vi "Multiple Analog Waveforms Output Generator LV2012.vi"() -> ()   [LabVIEW 2020]
uses:
  <vilib>/Utility/error.llb/DialogType.ctl
  <vilib>/DAQmx/write.llb/DAQmx Write (Analog 1D Wfm NChan NSamp).vi
  <vilib>/DAQmx/create/channels.llb/DAQmx Create Channel (AO-Voltage-Basic).vi
  <vilib>/DAQmx/configure/timing.llb/DAQmx Timing (Sample Clock).vi
  <vilib>/DAQmx/miscellaneous.llb/DAQmx Fill In Error Info.vi
  <resource>/objmgr/daqmx.rc
  <vilib>/measure/NI_MABase.lvlib
panel:
  in  "Phase (Deg)":dbl[](array[numeric])
  in  "Waveform Type":T1(array[ring])
  in  "Desired Frequency":dbl[](array[numeric]) caption="Desired Frequency (Hz)"
  in  "Amplitude":dbl[](array[numeric]) caption="Amplitude (V)"
  in  "Sample Clock Rate":dbl=10000.0 format="%.2f"
  in  "Samples per Buffer":dbl=1000.0
  in  "Physical Channels":tag="NI-USB6343/ao0:3"
  in  "Minimum Value":dbl=-10.0 format="%0.2f"
  in  "Maximum Value":dbl=10.0 format="%0.2f"
  out "Output Data":waveform(dbl)[](graph)
  in  "stop":bool
  # "Overview: This application demonstrates a method for generating multiple analog waveforms output on multiple channels. It also integrates a method for dynamically varying the output waveform attributes. All parameters including the waveform type, may be updated at run-time. This example is scalable to any number of available channels available on the system.\nRequirements: LabVIEW Full Developement System\nInstruction:\n1. Configure the physical channel.\n2. Configure the waveform attributes.\n3. Run the VI."
  # "DAQmx Task Configuration"
  # "Waveform Attributes"
  # "Introduction: \nThis application demonstrates a method\nfor generating multiple analog waveforms\noutput on multiple channels. It also integrates \na method for dynamically varying the output \nwaveform attributes. All parameters including \nthe waveform type, may be updated at run-\ntime. This example is scalable to any number \nof available channels."
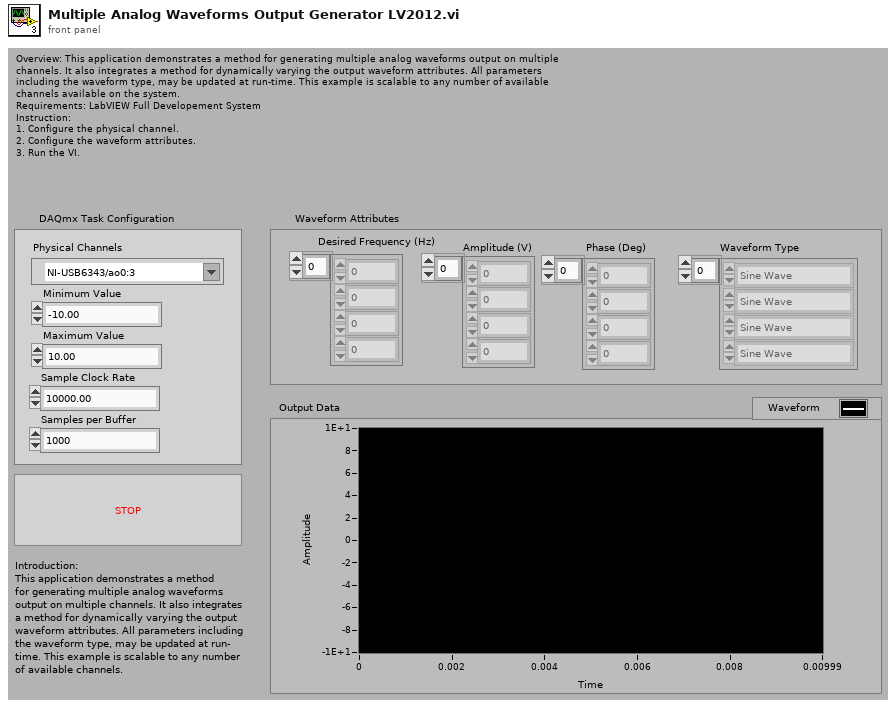
[diagram p1: front panel]
types:
  T1 = enum16{"Sine Wave", "Triangle Wave", "Square Wave", "Sawtooth Wave"}[]
  T2 = typedef "DialogType.ctl" = u16
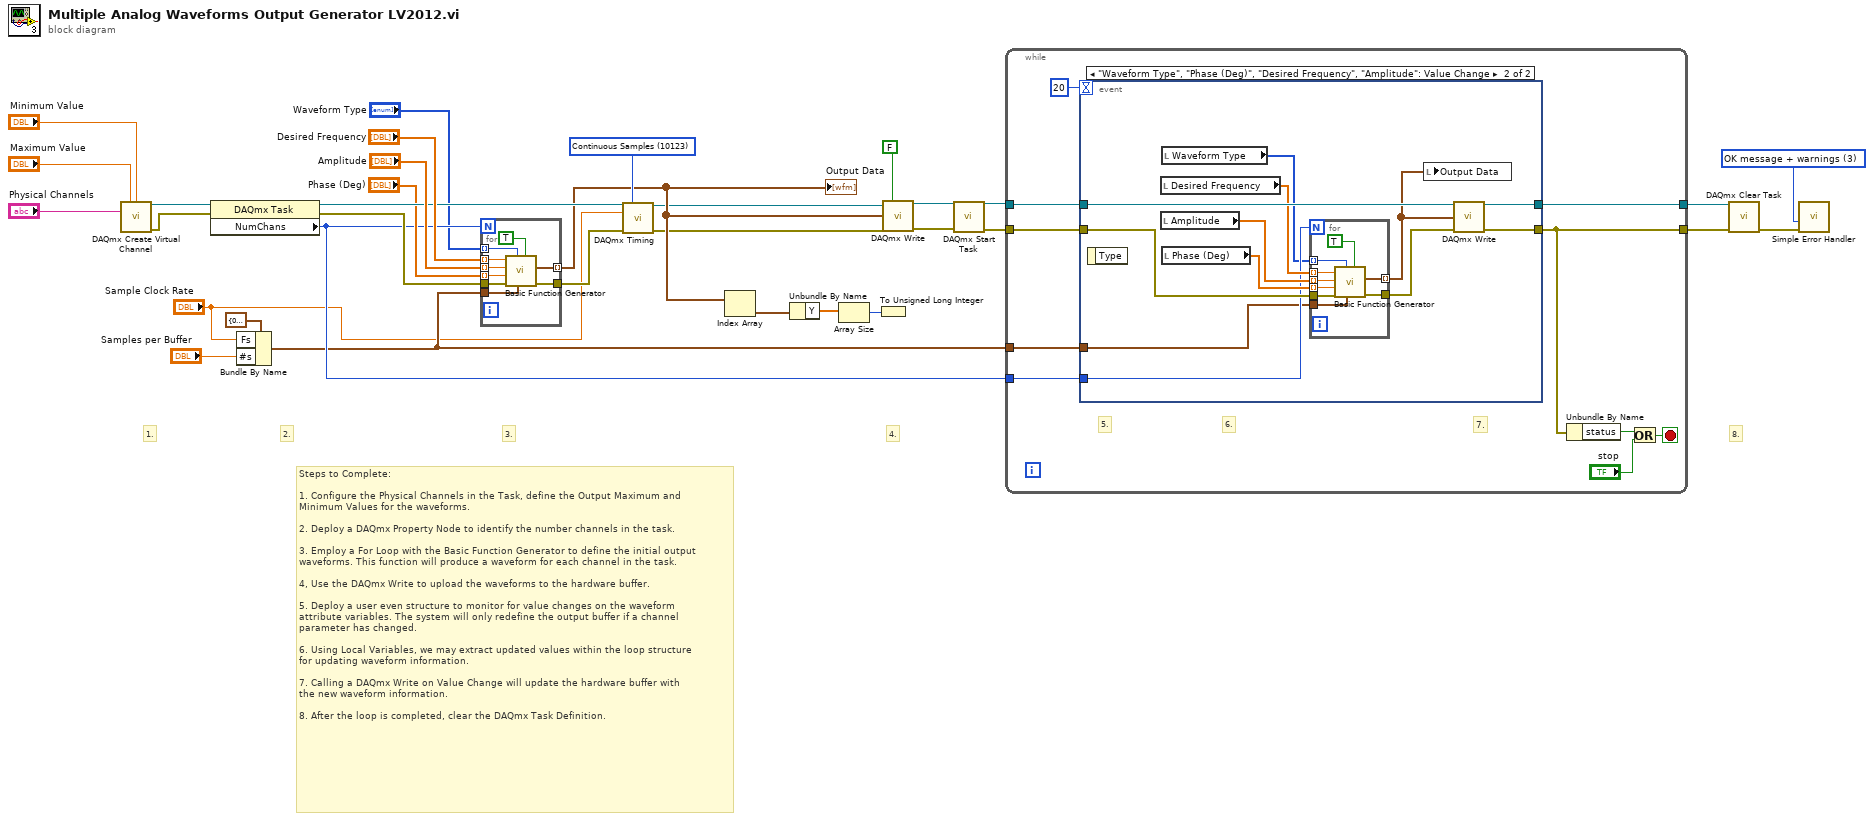
[diagram p0: block diagram]
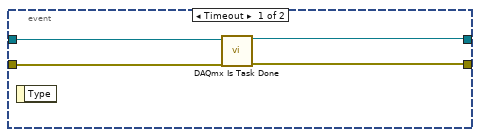
[diagram p2: hidden frame]
diagram:
  w24 = T2 3 items=["no dialog", "OK message", "continue or stop message", "OK message + warnings", "continue/stop + warnings"] ("type of dialog (OK msg:1)")
  w31 = 10123 items=["Finite Samples"=10178, "Continuous Samples"=10123] ("sample mode")
  # "Steps to Complete:\n\n1. Configure the Physical Channels in the Task, define the Output Maximum and \nMinimum Values for the waveforms. \n\n2. Deploy a DAQmx Property Node to identify the number channels in the task. \n\n3. Employ a For Loop with the Basic Function Generator to define the initial output\nwaveforms. This function will produce a waveform for each channel in the task. \n\n4, Use the DAQmx Write to upload the waveforms to the hardware buffer. \n\n5. Deploy a user even structure to monitor for value changes on the waveform \nattribute variables. The system will only redefine the output buffer if a channel \nparameter has changed. \n\n6. Using Local Variables, we may extract updated values within the loop structure\nfor updating waveform information. \n\n7. Calling a DAQmx Write on Value Change will update the hardware buffer with\nthe new waveform information. \n\n8. After the loop is completed, clear the DAQmx Task Definition."
  # "8."
  # "4."
  # "3."
  # "2."
  # "1."
  n1 = call-poly <vilib>:"DAQmx Create Virtual Channel.vi"("maximum value"="Maximum Value", "minimum value"="Minimum Value", "physical channels"="Physical Channels") -> ("task out"=w18:refnum<k21>, "error out"=w15:errorcluster)  [unwired: 11 in]
  n2 = property class="DAQmx Task"(reference=w18, error in=w15) -> (reference out=w17:refnum<k21>, error out=w16:errorcluster, "NumChans"=w13:u32)
  n3 = Bundle By Name(cluster=cluster{"Fs":dbl, "#s":dbl} {"Fs"=0.0, "#s"=0.0} ("sampling info"), "Fs"="Sample Clock Rate", "#s"="Samples per Buffer") -> (w9:cluster{"Fs":dbl, "#s":dbl})
  n4 = for {
    N: w13 -> [_]
    tunnel: "Amplitude" -> [w42] mode=indexing
    tunnel: "Desired Frequency" -> [w41] mode=indexing
    tunnel: [w40] -> w19
    tunnel: w16 -> [w39]
    tunnel: [w38] -> w6 mode=indexing
    tunnel: "Phase (Deg)" -> [w37] mode=indexing
    tunnel: w9 -> [w35]
    tunnel: "Waveform Type" -> [w34] mode=indexing
    n5 = call <vilib>:"Basic Function Generator.vi"("reset signal"=TRUE, "sampling info"=w35, "signal type"=w34, "error in (no error)"=w39, "phase"=w37, "amplitude"=w42, "frequency"=w41) -> ("error out"=w40:errorcluster, "signal out"=w38:waveform(dbl))  [unwired: 2 in, 1 out]
  }
  "Output Data" <- w6
  n6 = call-poly <vilib>:"DAQmx Timing.vi"("task/channels in"=w17, "sample mode"=w31, "rate"="Sample Clock Rate", "error in"=w19) -> ("task out"=w1:refnum<k21>, "error out"=w2:errorcluster)  [unwired: 10 in]
  n7 = Index Array(array=w6) -> (element=w5:waveform(dbl))  [unwired: 1 in]
  n8 = Unbundle By Name(w5) -> ("Y"=w4:dbl[])
  n9 = Array Size(array=w4) -> (size(s)=w3:i32)
  n10 = To Unsigned Long Integer(number=w3) -> ()  [unwired: 1 out]
  n11 = call-poly <vilib>:"DAQmx Write.vi"("task/channels in"=w1, "auto start"=FALSE, "data"=w6, "error in"=w2) -> ("task out"=w28:refnum<k21>, "error out"=w27:errorcluster)  [unwired: 9 in, 1 out]
  n12 = call <vilib>:"DAQmx Start Task.vi"("task/channels in"=w28, "error in"=w27) -> ("task out"=w32:refnum<k21>, "error out"=w26:errorcluster)  [unwired: 12 in]
  n13 = while {
    tunnel: w32 -> [w49]
    tunnel: w26 -> [w48]
    tunnel: w9 -> [w47]
    tunnel: w13 -> [w46]
    tunnel: [w45] -> w12
    tunnel: [w44] -> w11
    stop <- w51 stop-if-true
    # "7."
    # "6."
    # "5."
    n14 = event shown="[1] \"Waveform Type\", \"Phase (Deg)\", \"Desired Frequency\", \"Amplitude\": Value Change" {
      selector: _ -> [_ _]
      dyn-events: _ -> [_ _]
      timeout: 20 -> [_ _]
      tunnel: w49 -> [w56 w68]
      tunnel: w48 -> [w55 w67]
      tunnel: w47 -> [_ w58]
      tunnel: [w54 w62] -> w45
      tunnel: [w53 w61] -> w44
      tunnel: w46 -> [_ w59]
      event Timeout {
        n15 = event-data() -> ()  [unwired: 1 in, 1 out]
        n16 = call <vilib>:"DAQmx Is Task Done.vi"("task/channels in"=w56, "error in"=w55) -> ("task out"=w54:refnum<k21>, "error out"=w53:errorcluster)  [unwired: 11 in, 1 out]
      }
      event "Waveform Type", "Phase (Deg)", "Desired Frequency", "Amplitude": Value Change {
        n17 = event-data() -> ()  [unwired: 1 in, 1 out]
        n18 = local read "Desired Frequency"() -> (w65:dbl[])
        n19 = local read "Amplitude"() -> (w64:dbl[])
        n20 = local read "Waveform Type"() -> (w57:T1)
        n21 = local read "Phase (Deg)"() -> (w63:dbl[])
        n22 = for {
          N: w59 -> [_]
          tunnel: [w77] -> w66
          tunnel: [w76] -> w60 mode=indexing
          tunnel: w67 -> [w75]
          tunnel: w65 -> [w74] mode=indexing
          tunnel: w64 -> [w73] mode=indexing
          tunnel: w63 -> [w72] mode=indexing
          tunnel: w58 -> [w70]
          tunnel: w57 -> [w69] mode=indexing
          n23 = call <vilib>:"Basic Function Generator.vi"("reset signal"=TRUE, "sampling info"=w70, "signal type"=w69, "error in (no error)"=w75, "phase"=w72, "amplitude"=w73, "frequency"=w74) -> ("error out"=w77:errorcluster, "signal out"=w76:waveform(dbl))  [unwired: 2 in, 1 out]
        }
        n24 = local write "Output Data"(w60) -> ()
        n25 = call-poly <vilib>:"DAQmx Write.vi"("task/channels in"=w68, "data"=w60, "error in"=w66) -> ("task out"=w62:refnum<k21>, "error out"=w61:errorcluster)  [unwired: 10 in, 1 out]
      }
    }
    n26 = Unbundle By Name(w44) -> ("status"=w43:bool)
    n27 = Or(x=w43, y="stop") -> (x .or. y?=w51:bool)
  }
  n28 = call <vilib>:"DAQmx Clear Task.vi"("task in"=w12, "error in"=w11) -> ("error out"=w33:errorcluster)  [unwired: 13 in]
  n29 = call <vilib>:"Simple Error Handler.vi"("type of dialog (OK msg:1)"=w24, "error in (no error)"=w33) -> ()  [unwired: 3 in, 5 out]
